vi "Clear Buffer.vi"(0 "VISA resource name":refnum<visa-resource-name>, 5 "Buffer Name (defbuffer1)":string="defbuffer1", 11 "error in (no error)":errorcluster) -> (4 "VISA resource name out":refnum<visa-resource-name>, 15 "error out":errorcluster)   [LabVIEW 2024, in "Keithley 2450.lvlib"]
doc: "This clears the buffer data."
uses:
  C:/Users/Public/OneDrive/Desktop/Keithley_2450_2470_1_4_0_LV2015_NewReadme2_2450-LV2015-1.4.0/Keithley 2450/Keithley 2450.lvlib
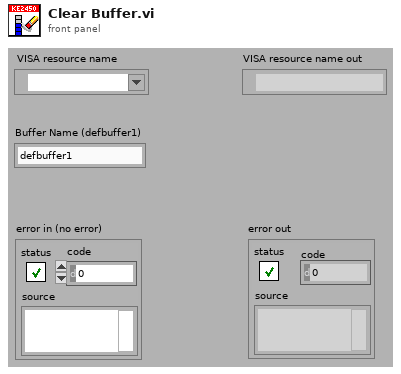
[diagram p1: front panel]
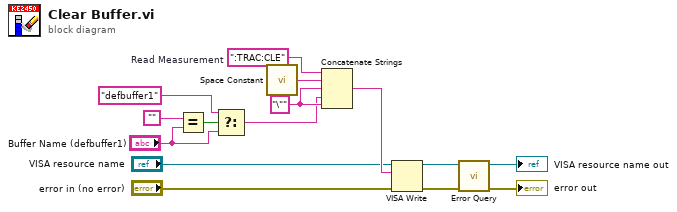
[diagram p0: block diagram]
diagram:
  w9 = "\""
  w6 = ":TRAC:CLE"  # Read Measurement
  n1 = Equal?(x="", y="Buffer Name (defbuffer1)") -> (x = y?=w12:bool)
  n2 = Select(t="defbuffer1", s=w12, f="Buffer Name (defbuffer1)") -> (s? t:f=w8:string)
  n3 = call <vilib>:"Space Constant.vi"() -> ("String"=w7:string)
  n4 = Concatenate Strings(w6, w7, w9, w8, w9) -> (w14:string)
  n5 = VISA Write(VISA resource name="VISA resource name", write buffer=w14, error in (no error)="error in (no error)") -> (VISA resource name out=w2:refnum<visa-resource-name>, error out=w1:errorcluster)  [unwired: 1 out]
  n6 = call "Error Query.vi"("error in (no error)"=w1, "VISA resource name"=w2) -> ("error out"=→"error out":errorcluster, "VISA resource name out"=→"VISA resource name out":refnum<visa-resource-name>)  [unwired: 8 out]
